vi "光敏.vi"() -> ()   [LabVIEW 2010]
uses:
  Instance           1 12Saved   光敏 .vi
  Instance           2 12Saved   光敏 .vi
  Instance           3 12Saved   光敏 .vi
  <vilib>/Analysis/NI_AALBase.lvlib
panel:
  in  "灵敏系数":dbl=40.0 format="%#.1f"
  out "电流（mA）":dbl(knob)=7.116224670410157 scale=0.0..10.0
  in  "stop":bool
  out "亮     度":bool
  in  "亮度调整":i32(slide)=100 scale=0.0..100.0
  # "光电传感器实验"
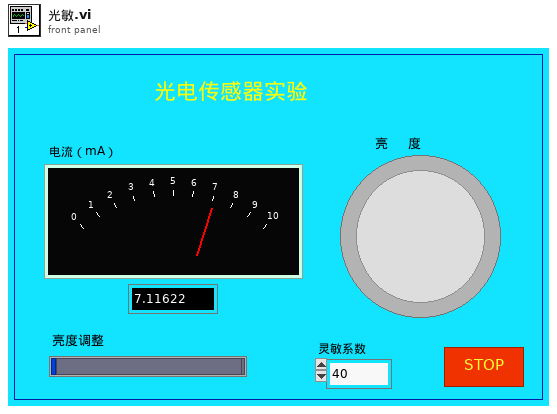
[diagram p1: front panel]
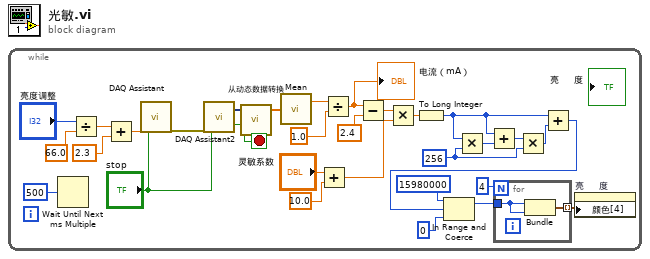
[diagram p0: block diagram]
diagram:
  n1 = while {
    stop <- w2 stop-if-true
    w31 = 256
    n2 = Wait Until Next ms Multiple(millisecond multiple=u32 500 ("毫秒倍数")) -> ()  [unwired: 1 out]
    n3 = Divide(x="亮度调整", y=66.0) -> (x/y=w22:dbl)
    n4 = Add(x=w22, y=2.3) -> (x+y=w10:dbl)
    n5 = call "DAQ Assistant"("data"=w10, "stop (T)"="stop") -> ("error out"=w7:errorcluster)  [unwired: 16 in, 1 out]
    n6 = call "DAQ Assistant2"("error in"=w7, "stop (F)"="stop") -> ("data"=w9:dynamicdata, "stopped"=w2:bool)  [unwired: 14 in, 2 out]
    n7 = call "从动态数据转换"("Dynamic Data Type"=w9) -> ("Array"=w6:dbl[])  [unwired: 3 in]
    n8 = call <vilib>:"Mean.vi"("X"=w6) -> ("mean"=w5:dbl)  [unwired: 1 out]
    n9 = Add(x="灵敏系数", y=10.0) -> (x+y=w12:dbl)
    n10 = Divide(x=w5, y=1.0) -> (x/y=w4:dbl)
    "电流（mA）" <- w4
    n11 = Subtract(x=w4, y=2.4) -> (x-y=w21:dbl)
    n12 = Multiply(x=w21, y=w12) -> (x*y=w18:dbl)
    n13 = To Long Integer(number=w18) -> (32bit integer=w16:i32)
    n14 = Multiply(x=w16, y=w31) -> (x*y=w19:i32)
    n15 = Add(x=w16, y=w19) -> (x+y=w30:i32)
    n16 = Multiply(x=w30, y=w31) -> (x*y=w17:i32)
    n17 = Add(x=w16, y=w17) -> (x+y=w29:i32)
    n18 = In Range and Coerce(upper limit=15980000, x=w29, lower limit=0) -> (coerced(x)=w15:i32)  [unwired: 1 out]
    n19 = for {
      N: 4 -> [_]
      tunnel: w15 -> [w33]
      tunnel: [w32] -> w27 mode=indexing
      n20 = Bundle("upper limit"=w33, "upper limit"=w33) -> (w32:cluster{"upper limit":i32, "upper limit":i32})  [unwired: 1 in]
    }
    n21 = property on="亮     度" class="Bool (严格)"("颜色[4]"=w27) -> ()  [unwired: 2 in, 2 out]
  }
